vi "Acroname_All_Ports_Enable.vi"(8 "error in (no error)":errorcluster) -> (0 "error out":errorcluster, 2 "Ports Failed":i32[](array[numeric]), 3 "Successful?":bool)   [LabVIEW 2025]
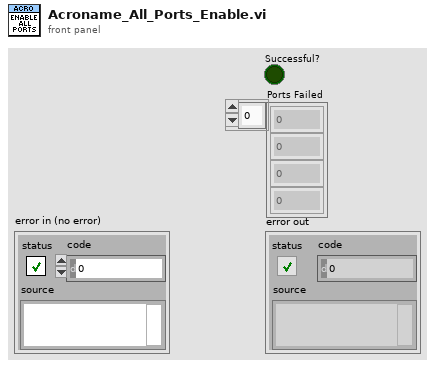
[diagram p1: front panel]
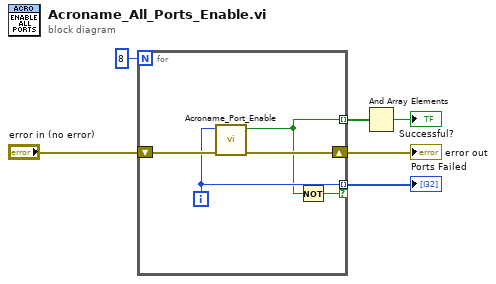
[diagram p0: block diagram]
diagram:
  n1 = for {
    N: 8 -> [_]
    tunnel: [w8] -> w3 mode=indexing
    shift-right: [w10] -> w4
    shift-left: "error in (no error)" -> [w11]
    tunnel: [w9] -> w1 mode=indexing if=w7
    i -> [w9]
    n2 = call "Acroname_Port_Enable.vi"("error in (no error)"=w11, "Port Number"=w9) -> ("error out"=w10:errorcluster, "Enable Successful?"=w8:bool)  [unwired: 6 in, 2 out]
    n3 = Not(x=w8) -> (.not. x?=w7:bool)
  }
  "error out" <- w4
  "Ports Failed" <- w1
  n4 = And Array Elements(Boolean array=w3) -> (logical AND=→"Successful?":bool)
